vi "DCS(Upgrade).vi"(3 "error in":errorcluster) -> (10 "error out":errorcluster)   [LabVIEW 2013]
uses:
  <userlib>/Accelerator/User Interface/Controls/dcs points.ctl
  <userlib>/Accelerator/User Interface/Controls/dcs_spot.ctl
  <vilib>/gmath/NI_Gmath.lvlib
  <vilib>/Utility/miscctls.llb/LVPointTypeDef.ctl
  <vilib>/gmath/NumericalOptimization/Nonlinear Curve Fit LM.vi
  <userlib>/Accelerator/User Interface/Controls/Role ID.ctl
panel:
  in  "Waveform Path":path=path "C:/Users/Chris/Desktop/DCS(Upgrade)/Waveforms"
  in  "Nornamiled":path=path "C:/Users/Chris/Desktop/DCS(Upgrade)/dcs_data/dcs_normalized.csv"
  in  "XY and Max":path=path "C:/Users/Chris/Desktop/DCS(Upgrade)/dcs_points/dcs_points.csv"
  in  "Points to Check Noise":i32=2000
  in  "Color bar Control":cluster{dbl, u32}[](array[cluster])
  in  "stop":bool
  in  "Tab Control":T1(tab)
  out "Intensity Graph":dbl[][](graph)
  in  "Spot Save Folder":path=path "C:/Users/Chris/Desktop/DCS(Upgrade)/dcs_data"
  in  "Save Spot Image":bool
  in  "Clear Spot/Track":bool
  in  "Particle Limit":i64=500 min=0 step=10
  out "Laser spot\nMove (mm)":dbl[](array[numeric])=[nan, nan] format="%#.3g"
  out "Avg. Freq. (Hz)":dbl
  in  "Orange Cursor Position":dbl[](array[numeric])=[0.0, 0.0] min=-12.0 max=12.0 step=0.1 format="%.3g"
  out "Spot Widths":dbl[](array[numeric]) format="%.6g"
  out "Countdown to\nnext track point":i32=1
  out "XY Graph":cluster{"Y":dbl[], "Y":dbl[]}[](graph)
  in  "Load old position\nto Orange Cursor":bool
  in  "Set Orange Cursor\nto current position":bool
  out "# of Particles\nin Spot":dbl
  out "Current Spot Pos":dbl[](array[numeric])=[nan, nan] format="%.3g"
  in  "# of shots to calculate spot":i32=20
  out "Spot Size over time":dbl[][](graph)
  out "Filtered Signals":dbl[][](graph)
  out "Unfiltered Signals":ext[][](graph)
  in  "Record Normalized":bool
  in  "Record XY":bool
  in  "External Trigger":bool
  in  "Auto Threshold":bool
  out "Sampling Frequency":u16(ring) items=["40 MHz", "20 MHz", "10 MHz", "5 MHz", "2.5 MHz", "1 MHz", "100 kHz", "10 kHz"]
  out "Length of Sample":dbl caption="s" format="%^#_3g"
  out "Memory Address Pointer":ext
  out "Post trigger Size":ext
  out "Pretrigger Size":ext
  out "Trigger Generation register":i32=23 format="%.0b"
  out "status register":i8=4 format="%08b"
  out "control register":i16=23 format="%015b"
  in  "Posttrigger size":i32
  in  "Acquisition Rate":u16(ring) items=["40 MHz", "20 MHz", "10 MHz", "5 MHz", "2.5 MHz", "1 MHz", "100 kHz", "10 kHz"]
  in  "Pretrigger size":i32=1000
  in  "Rising or falling?":bool
  out "Running Errors":errorcluster
  in  "Jorger TR slot":i32=3
  in  "Timeout (# of Cycles)":i32=100
  in  "Channels":i32[](array[numeric])=[0, 1, 2, 3, 4, 5, 6, 7]
  in  "Median Filter Rank":i32=30
  in  "Thresholds":ext[](array[numeric])
  in  "Level Buffer":i32=25
  # "DAQ Parameter Indicators"
  # "DAQ Parameter Controls"
  # "Falling"
  # "Rising"
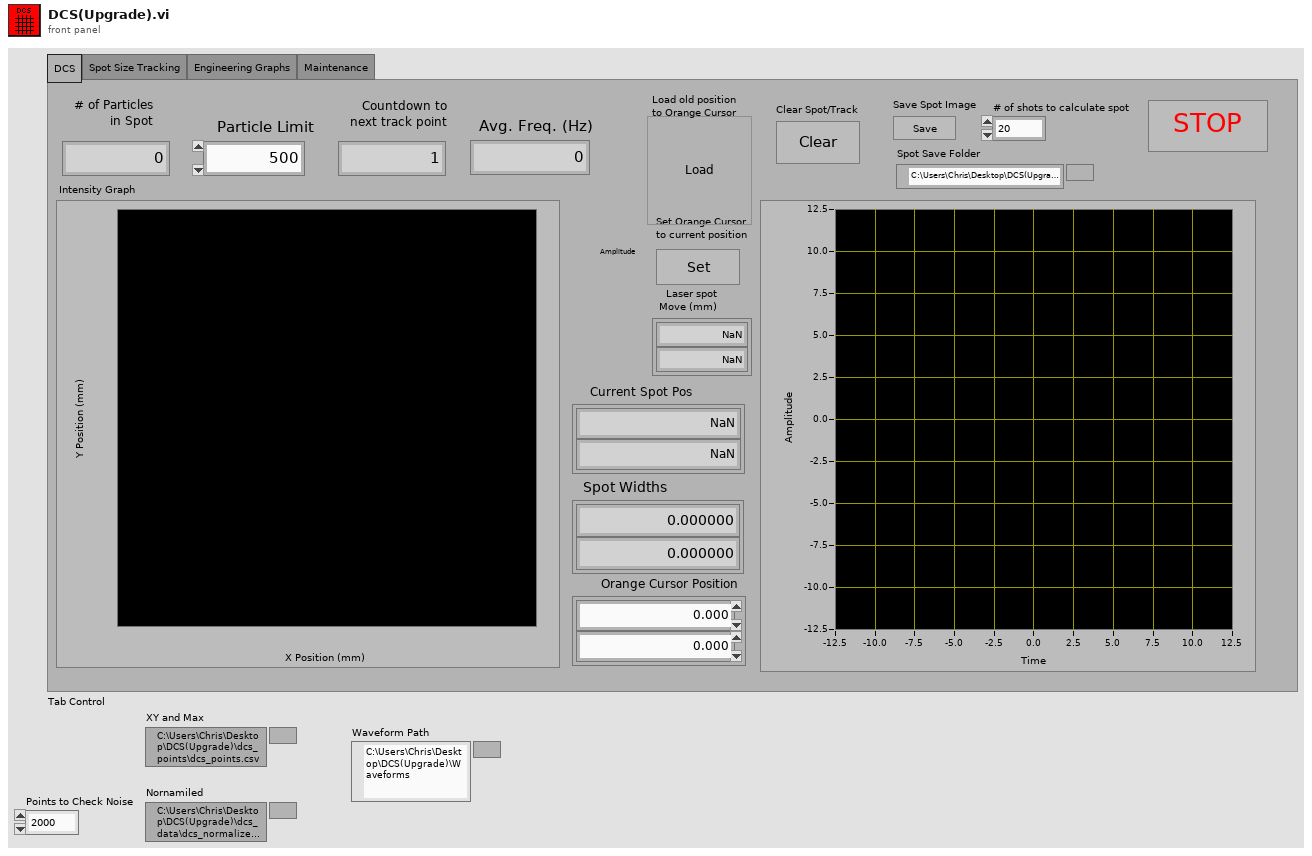
[diagram p1: front panel]
types:
  T1 = enum32{"DCS", "Spot Size Tracking", "Engineering Graphs", "Maintenance"}
  T2 = typedef "LVPointTypeDef.ctl" = cluster{"Horizontal":i16, "Vertical":i16}
  T3 = typedef "dcs_spot.ctl" = cluster{"DCS spot ID":i32, "Integer Timestamp":i64, "Spot X":dbl, "Spot Y":dbl, "Spot Width X":dbl, "Spot Width Y":dbl, "Spot Size":i32, "Experiment Settings ID":i32}
  T4 = typedef "Role ID.ctl" = enum16{"First_Detector", "Second_Detector", "Third_Detector", "LeCroy_CH1", "LeCroy_CH2", "LeCroy_CH3", "LeCroy_CH4", "PSU", "DCS 1", "DCS 2"}
  T5 = cluster{"Data":dbl[][], "Integer Timestamp":u64, "Signal Length":u32, "DCS_ID":u64, "Role ID":T4}
  T6 = typedef "dcs points.ctl" = cluster{"Integer Timestamp":i64, "X":dbl, "Y":dbl, "DCS spot ID":i32}
  T7 = cluster{"Data":dbl[][], "Integer Timestamp":u64, "Signal Length":u32, "DCS_ID":u64, "Role ID":T4}[]
  T8 = typedef "imagedata.ctl" = cluster{"image type":i32, "image depth":i32, "image":u8[], "mask":u8[], "colors":u32[], "Rectangle":cluster{"left":i16, "top":i16, "right":i16, "bottom":i16}}
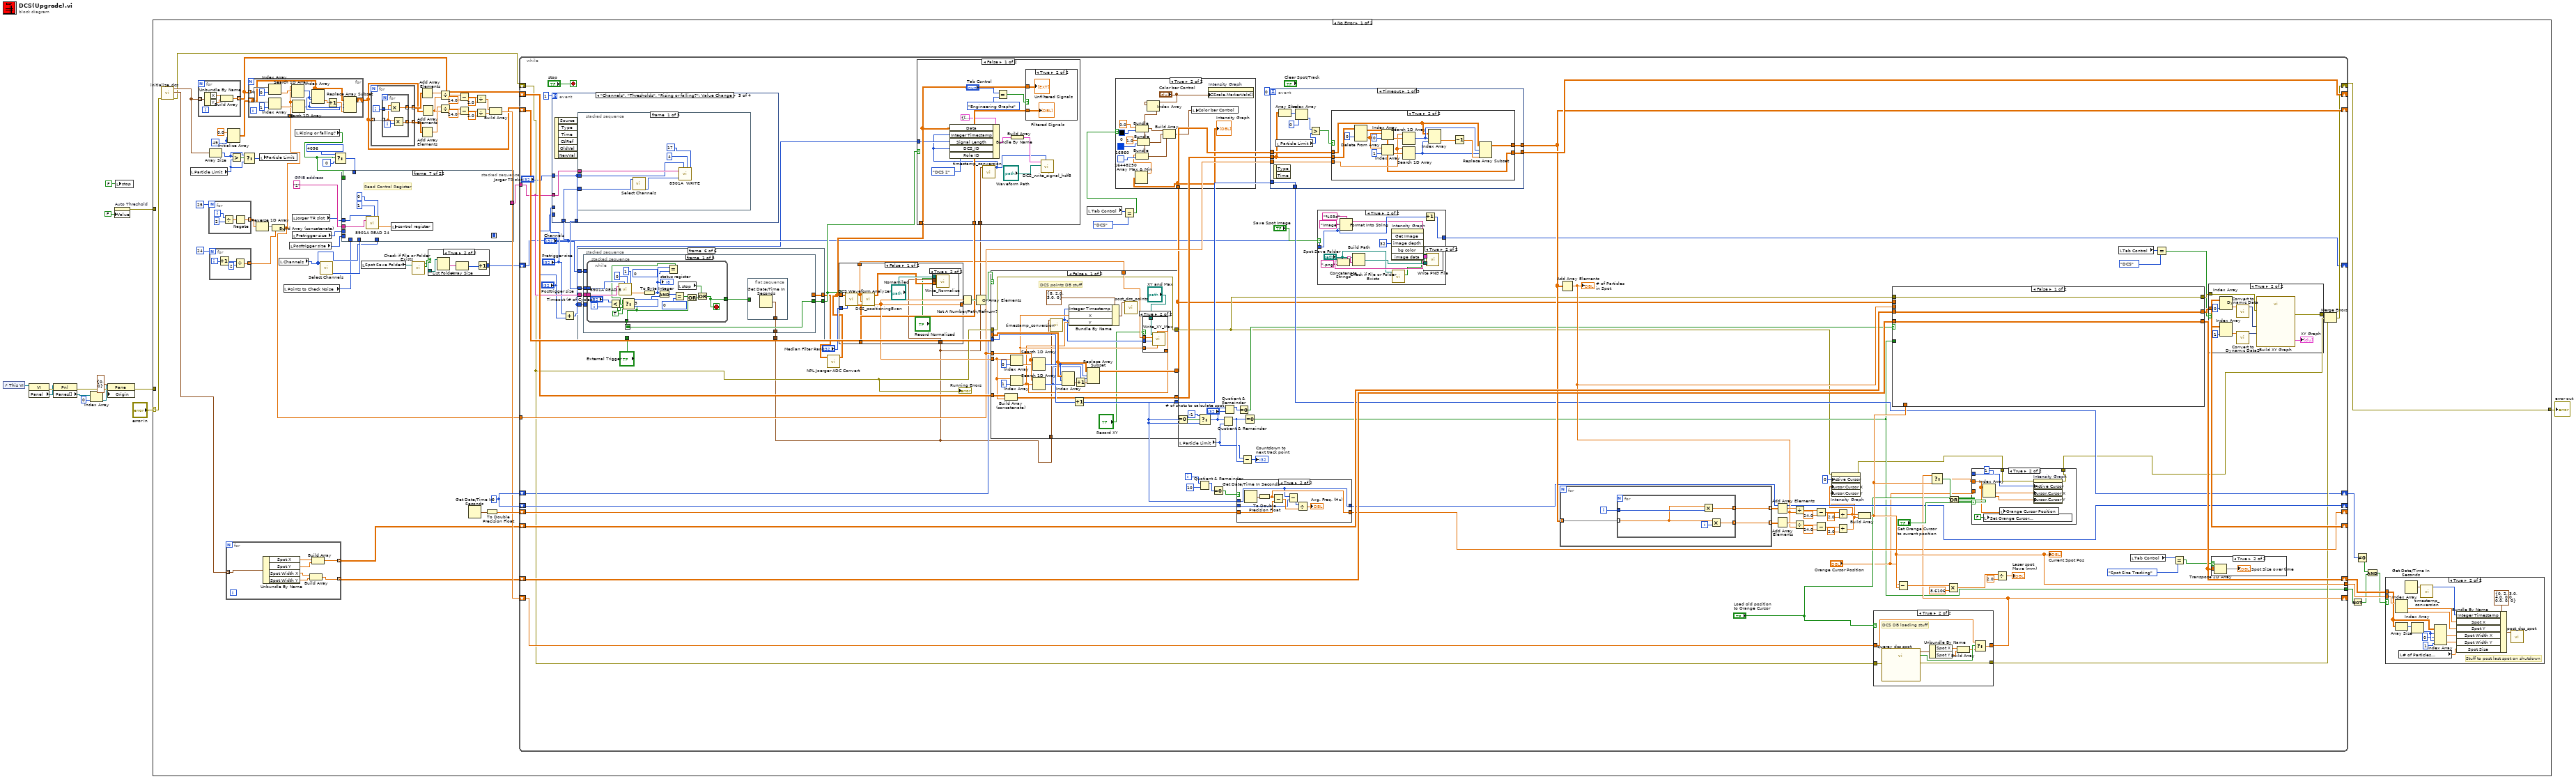
[diagram p0: block diagram]
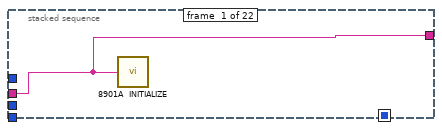
[diagram p2: hidden frame]
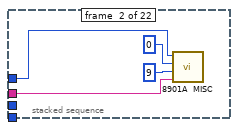
[diagram p3: hidden frame]
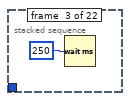
[diagram p4: hidden frame]
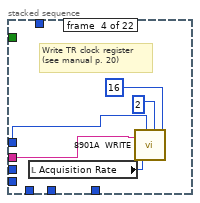
[diagram p5: hidden frame]
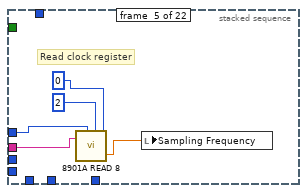
[diagram p6: hidden frame]
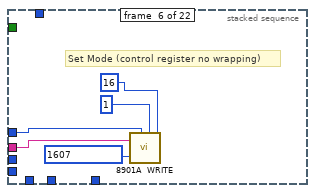
[diagram p7: hidden frame]
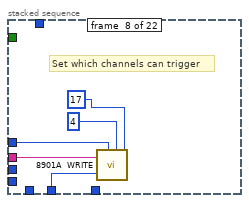
[diagram p8: hidden frame]
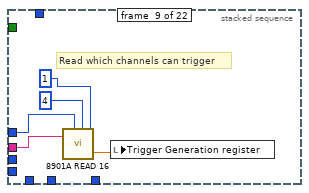
[diagram p9: hidden frame]
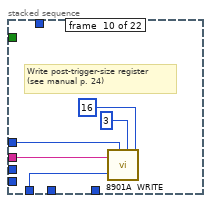
[diagram p10: hidden frame]
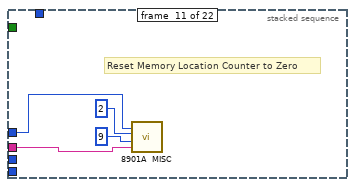
[diagram p11: hidden frame]
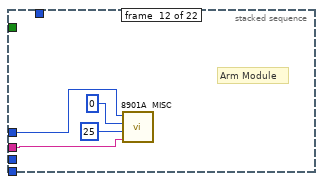
[diagram p12: hidden frame]
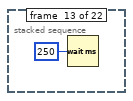
[diagram p13: hidden frame]
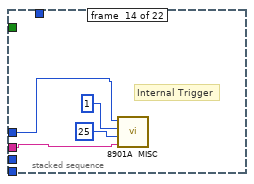
[diagram p14: hidden frame]
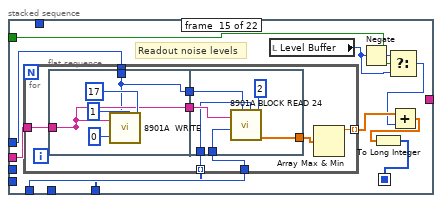
[diagram p15: hidden frame]
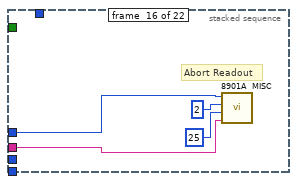
[diagram p16: hidden frame]
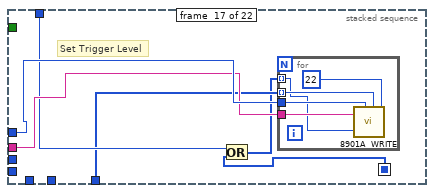
[diagram p17: hidden frame]
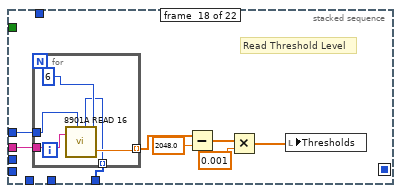
[diagram p18: hidden frame]
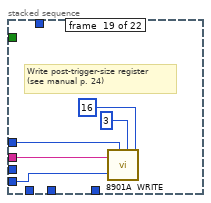
[diagram p19: hidden frame]
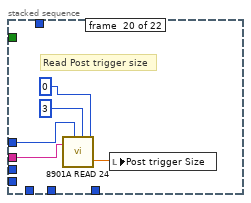
[diagram p20: hidden frame]
diagram:
  n1 = control-ref of="This VI"() -> (w11:refnum<vi>)
  n2 = property class="VI"(reference=w11) -> (error out=w10:errorcluster, "Panel"=w9:refnum<vi>)  [unwired: 1 in, 1 out]
  n3 = property class="Pnl"(reference=w9, error in=w10) -> (error out=w8:errorcluster, "Panes[]"=w7:refnum<vi>[])  [unwired: 1 out]
  n4 = Index Array(array=w7, index=0) -> (element=w5:refnum<vi>)
  n5 = property class="Pane"(reference=w5, error in=w8, "Origin"=T2 {"Horizontal"=0, "Vertical"=0}) -> (error out=w3:errorcluster)  [unwired: 1 out]
  n6 = property on="Auto Threshold" class="Bool (strict)"("Value"=FALSE ("Auto Threshold")) -> (error out=w1:errorcluster)  [unwired: 2 in, 1 out]
  n7 = local write "stop"(FALSE ("stop")) -> ()
  n8 = case shown="No Error" "error in" {
    selector: "error in" -> [w33 w956]
    tunnel: [w32 w956] -> w13
    tunnel: w3 -> [_ _]
    tunnel: w1 -> [_ _]
    frame No Error {
      w26 = "2"  # GPIB address
      w53 = 49 ("dimension size")
      w56 = 0
      n9 = call <userlib>:"initialize_dcs.vi"("error in (no error)"=w33) -> ("error out"=w27:errorcluster, "Dust Spot Array"=w45:T3[], "Dust Point Array"=w38:T6[])  [unwired: 8 in]
      n10 = local read "Particle Limit"() -> (w35:i64)
      n11 = for {
        tunnel: [w236] -> w44 mode=indexing
        tunnel: w38 -> [w235] mode=indexing
        n12 = Unbundle By Name(w235) -> ("X"=w238:dbl, "Y"=w237:dbl)
        n13 = Build Array(w238, w237) -> (w236:dbl[])
      }
      n14 = for {
        N: 25 -> [_]
        tunnel: [w267] -> w76 mode=indexing
        i -> [w270]
        n15 = Divide(x=w270, y=2) -> (x/y=w268:dbl)
        n16 = Negate(x=w268) -> (-x=w267:dbl)
      }
      n17 = Array Size(array=w38) -> (size(s)=w36:i32)
      n18 = for {
        N: 24 -> [_]
        tunnel: [w264] -> w74 mode=indexing
        i -> [w266]
        n19 = Increment(x=w266) -> (x+1=w263:i32)
        n20 = Divide(x=w263, y=2) -> (x/y=w264:dbl)
      }
      n21 = for {
        tunnel: [w230] -> w48 mode=indexing
        tunnel: [w229] -> w49 mode=indexing
        tunnel: w45 -> [w228] mode=indexing
        n22 = Unbundle By Name(w228) -> ("Spot X"=w234:dbl, "Spot Y"=w233:dbl, "Spot Width X"=w232:dbl, "Spot Width Y"=w231:dbl)
        n23 = Build Array(w232, w231) -> (w230:dbl[])
        n24 = Build Array(w234, w233) -> (w229:dbl[])
      }
      n25 = Initialize Array(0.0 ("element"), w53, w53) -> (w52:dbl[][])
      n26 = Greater?(x=w36, y=w35) -> (0:w37:bool)
      n27 = Select(t=w36, s=w37, f=w35) -> (s? t:f=w34:i64)
      n28 = Reverse 1D Array(array=w76) -> (reversed array=w75:dbl[])
      n29 = local write "Particle Limit"(w34) -> ()
      n30 = Build Array (concatenate)(w75, w74) -> (w50:dbl[])
      n31 = for {
        tunnel: w44 -> [w225] mode=indexing
        tunnel: w50 -> [w216]
        shift-right: [w217] -> w43
        shift-left: w52 -> [w218]
        n32 = Index Array(array=w225, index=0) -> (element=w224:dbl)
        n33 = Index Array(array=w225, index=1) -> (element=w223:dbl)
        n34 = Search 1D Array(1D array=w216, element=w224) -> (index of element=w220:i32)  [unwired: 1 in]
        n35 = Search 1D Array(1D array=w216, element=w223) -> (index of element=w219:i32)  [unwired: 1 in]
        n36 = Index Array(array=w218, index (row)=w220, index (col)=w219) -> (element=w222:dbl)
        n37 = Increment(x=w222) -> (x+1=w221:dbl)
        n38 = Replace Array Subset(array=w218, new element=w221, index (row)=w220, index (col)=w219) -> (w217:dbl[][])
      }
      n39 = local read "Channels"() -> (w17:i32[])
      n40 = local read "Points to Check Noise"() -> (w16:i32)
      n41 = local read "Posttrigger size"() -> (w22:i32)
      n42 = local read "Jorger TR slot"() -> (w24:i32)
      n43 = local read "Pretrigger size"() -> (w23:i32)
      n44 = local read "Rising or falling?"() -> (w15:bool)
      n45 = call <userlib>:"Select Channels.vi"("Channels"=w17) -> ("Channels in Use"=w21:u32)  [unwired: 10 in]
      n46 = Select(t=4096, s=w15, f=0) -> (s? t:f=w18:i32)
      n47 = stacked-sequence {
        seq-local: [_ _ _ _ _ _ _ _ _ _ _ _ _ _ w137 _ _ _ _ _ _ _] -> [_ _ _ _ _ _ _ _ _ _ _ _ _ _ _ _ w167 _ _ _ _ _]
        tunnel: w24 -> [_ w80 _ w87 w92 w95 w102 w106 w111 w117 w121 w124 _ w129 w139 w164 w172 w185 w193 w198 w203 w208]
        tunnel: w26 -> [w79 w81 _ w86 w91 w96 w101 w107 w112 w116 w120 w125 _ w130 w143 w163 w171 w184 w192 w197 w202 w207]
        tunnel: w23 -> [_ _ _ _ _ _ _ _ _ _ _ _ _ _ _ _ _ _ _ _ w201 _]
        tunnel: w22 -> [_ _ _ _ _ _ _ _ _ _ _ _ _ _ _ _ _ _ w191 _ _ _]
        tunnel: [w79 _ _ _ _ _ _ _ _ _ _ _ _ _ _ _ _ _ _ _ _ _] -> w25
        tunnel: w21 -> [_ _ _ _ _ _ _ w105 _ _ _ _ _ _ _ _ _ _ _ _ _ _]
        tunnel: w16 -> [_ _ _ _ _ _ _ _ _ w115 _ _ _ _ w142 _ _ _ _ _ _ _]
        tunnel: w18 -> [_ _ _ _ _ _ _ _ _ _ _ _ _ _ _ _ w170 _ _ _ _ _]
        tunnel: w17 -> [_ _ _ _ _ _ _ _ _ _ _ _ _ _ w140 _ w169 w179 _ _ _ _]
        tunnel: w15 -> [_ _ _ _ _ _ _ _ _ _ _ _ _ _ w134 _ _ _ _ _ _ _]
        frame #0 {
          n48 = call <instrlib>:"8901A  INITIALIZE.vi"("GPIB address"=w79) -> ()
        }
        frame #1 {
          n49 = call <instrlib>:"8901A  MISC.vi"("GPIB address"=w81, "f"=9, "a"=0, "n"=w80) -> ()
        }
        frame #2 {
          n50 = Wait (ms)(milliseconds to wait=250) -> ()  [unwired: 1 out]
        }
        frame #3 {
          # "Write TR clock register\n(see manual p. 20)"
          n51 = local read "Acquisition Rate"() -> (w85:u16)
          n52 = call <instrlib>:"8901A  WRITE.vi"("data"=w85, "GPIB address"=w86, "n"=w87, "a"=2, "f"=16) -> ()  [unwired: 1 in]
        }
        frame #4 {
          # "Read clock register"
          n53 = call <instrlib>:"8901A READ 8.vi"("GPIB address"=w91, "n"=w92, "a"=2, "f"=0) -> ("output"=w90:ext)  [unwired: 3 in]
          n54 = local write "Sampling Frequency"(w90) -> ()
        }
        frame #5 {
          # "Set Mode (control register no wrapping)"
          n55 = call <instrlib>:"8901A  WRITE.vi"("data"=1607, "GPIB address"=w96, "n"=w95, "a"=1, "f"=16) -> ()  [unwired: 1 in]
        }
        frame #6 {
          # "Read Control Register"
          n56 = call <instrlib>:"8901A READ 24.vi"("GPIB address"=w101, "n"=w102, "a"=1, "f"=0) -> ("output"=w100:ext)  [unwired: 3 in]
          n57 = local write "control register"(w100) -> ()
        }
        frame #7 {
          # "Set which channels can trigger"
          n58 = call <instrlib>:"8901A  WRITE.vi"("data"=w105, "GPIB address"=w107, "n"=w106, "a"=4, "f"=17) -> ()  [unwired: 1 in]
        }
        frame #8 {
          # "Read which channels can trigger"
          n59 = call <instrlib>:"8901A READ 16.vi"("GPIB address"=w112, "n"=w111, "a"=u8 4, "f"=u8 1) -> ("output"=w110:ext)  [unwired: 3 in]
          n60 = local write "Trigger Generation register"(w110) -> ()
        }
        frame #9 {
          # "Write post-trigger-size register\n(see manual p. 24)"
          n61 = call <instrlib>:"8901A  WRITE.vi"("data"=w115, "GPIB address"=w116, "n"=w117, "a"=3, "f"=16) -> ()  [unwired: 1 in]
        }
        frame #10 {
          # "Reset Memory Location Counter to Zero"
          n62 = call <instrlib>:"8901A  MISC.vi"("GPIB address"=w120, "f"=u8 9, "a"=u8 2, "n"=w121) -> ()
        }
        frame #11 {
          # "Arm Module"
          n63 = call <instrlib>:"8901A  MISC.vi"("GPIB address"=w125, "f"=25, "a"=0, "n"=w124) -> ()
        }
        frame #12 {
          n64 = Wait (ms)(milliseconds to wait=u32 250) -> ()  [unwired: 1 out]
        }
        frame #13 {
          # "Internal Trigger"
          n65 = call <instrlib>:"8901A  MISC.vi"("GPIB address"=w130, "f"=u8 25, "a"=u8 1, "n"=w129) -> ()
        }
        frame #14 {
          # "Readout noise levels"
          n66 = for {
            tunnel: w143 -> [w150]
            tunnel: w142 -> [w149]
            tunnel: [w147] -> w141 mode=indexing
            tunnel: w140 -> [w146] mode=indexing
            tunnel: w139 -> [w145]
            n67 = flat-sequence {
              tunnel: [w154] -> _
              tunnel: [w154] -> w151
              tunnel: w150 -> [w154]
              tunnel: w145 -> [w152]
              tunnel: [w152] -> w144
              tunnel: w151 -> [w161]
              tunnel: [w160] -> w148
              tunnel: w149 -> [w159]
              tunnel: w146 -> [w158]
              tunnel: w144 -> [w157]
              frame #0 {
                n68 = call <instrlib>:"8901A  WRITE.vi"("data"=0, "GPIB address"=w154, "n"=w152, "a"=1, "f"=17) -> ()  [unwired: 1 in]
              }
              frame #1 {
                n69 = call <instrlib>:"8901A BLOCK READ 24.vi"("f"=2, "a"=w158, "n"=w157, "GPIB address"=w161, "# points to read"=w159) -> ("output"=w160:ext[])  [unwired: 4 in]
              }
            }
            n70 = Array Max & Min(array=w148) -> (max value=w147:ext)  [unwired: 3 out]
          }
          n71 = local read "Level Buffer"() -> (w136:i32)
          n72 = Negate(x=w136) -> (-x=w135:i32)
          n73 = Select(t=w135, s=w134, f=w136) -> (s? t:f=w133:i32)
          n74 = Add(x=w141, y=w133) -> (x+y=w138:ext[])
          n75 = To Long Integer(number=w138) -> (32bit integer=w137:i32[])
        }
        frame #15 {
          # "Abort Readout"
          n76 = call <instrlib>:"8901A  MISC.vi"("GPIB address"=w163, "f"=25, "a"=2, "n"=w164) -> ()
        }
        frame #16 {
          # "Set Trigger Level"
          n77 = Or(x=w170, y=w167) -> (x .or. y?=w168:i32[])
          n78 = for {
            tunnel: w172 -> [w176]
            tunnel: w171 -> [w175]
            tunnel: w169 -> [w174] mode=indexing
            tunnel: w168 -> [w173] mode=indexing
            n79 = call <instrlib>:"8901A  WRITE.vi"("data"=w173, "GPIB address"=w175, "n"=w176, "a"=w174, "f"=u8 22) -> ()  [unwired: 1 in]
          }
        }
        frame #17 {
          # "Read Threshold Level"
          n80 = for {
            tunnel: w185 -> [w189]
            tunnel: w184 -> [w188]
            tunnel: [w187] -> w182 mode=indexing
            tunnel: w179 -> [w186] mode=indexing
            n81 = call <instrlib>:"8901A READ 16.vi"("GPIB address"=w188, "n"=w189, "a"=w186, "f"=u8 6) -> ("output"=w187:ext)  [unwired: 3 in]
          }
          n82 = Subtract(x=w182, y=2048.0) -> (x-y=w180:ext[])
          n83 = Multiply(x=w180, y=0.001) -> (x*y=w178:ext[])
          n84 = local write "Thresholds"(w178) -> ()
        }
        frame #18 {
          # "Write post-trigger-size register\n(see manual p. 24)"
          n85 = call <instrlib>:"8901A  WRITE.vi"("data"=w191, "GPIB address"=w192, "n"=w193, "a"=3, "f"=16) -> ()  [unwired: 1 in]
        }
        frame #19 {
          # "Read Post trigger size"
          n86 = call <instrlib>:"8901A READ 24.vi"("GPIB address"=w197, "n"=w198, "a"=3, "f"=0) -> ("output"=w196:ext)  [unwired: 3 in]
          n87 = local write "Post trigger Size"(w196) -> ()
        }
        frame #20 {
          # "Write Pretrigger size"
          n88 = call <instrlib>:"8901A  WRITE.vi"("data"=w201, "GPIB address"=w202, "n"=w203, "a"=4, "f"=16) -> ()  [unwired: 1 in]
        }
        frame #21 {
          # "Read Pretrigger size"
          n89 = call <instrlib>:"8901A READ 16.vi"("GPIB address"=w207, "n"=w208, "a"=u8 4, "f"=u8 0) -> ("output"=w206:ext)  [unwired: 3 in]
          n90 = local write "Pretrigger Size"(w206) -> ()
        }
      }
      n91 = local read "Spot Save Folder"() -> (w30:path)
      n92 = for {
        tunnel: w43 -> [w257] mode=indexing
        tunnel: [w255] -> w73 mode=indexing
        tunnel: [w254] -> w72 mode=indexing
        i -> [w256]
        n93 = for {
          tunnel: w257 -> [w259] mode=indexing
          tunnel: w256 -> [w262]
          tunnel: [w260] -> w254 mode=indexing
          tunnel: [w258] -> w255 mode=indexing
          i -> [w261]
          n94 = Multiply(x=w259, y=w262) -> (x*y=w258:dbl)
          n95 = Multiply(x=w259, y=w261) -> (x*y=w260:dbl)
        }
      }
      n96 = call <vilib>:"Check if File or Folder Exists.vi"("path"=w30) -> ("file or folder exists?"=w29:bool, "dup path"=w28:path)  [unwired: 8 in, 1 out]
      n97 = Add Array Elements(numeric array=w73) -> (sum=w71:dbl)
      n98 = Add Array Elements(numeric array=w72) -> (sum=w70:dbl)
      n99 = Add Array Elements(numeric array=w43) -> (sum=w62:dbl)
      n100 = case shown="True" w29 {
        tunnel: [0 w213] -> w31
        tunnel: w28 -> [_ w212]
        frame False {
        }
        frame True {
          n101 = List Folder(path=w212) -> (filenames=w215:string[])  [unwired: 3 in, 3 out]
          n102 = Array Size(array=w215) -> (size(s)=w214:i32)
          n103 = Increment(x=w214) -> (x+1=w213:i32)
        }
      }
      n104 = Divide(x=w71, y=w62) -> (x/y=w69:dbl)
      n105 = Divide(x=w70, y=w62) -> (x/y=w68:dbl)
      n106 = Subtract(x=w69, y=24.0) -> (x-y=w60:dbl)
      n107 = Subtract(x=w68, y=24.0) -> (x-y=w66:dbl)
      n108 = Get Date/Time In Seconds() -> (seconds since 1Jan1904=w58:timestamp)
      n109 = Divide(x=w60, y=2.0) -> (x/y=w59:dbl)
      n110 = Divide(x=w66, y=2.0) -> (x/y=w63:dbl)
      n111 = To Double Precision Float(number=w58) -> (double precision float=w57:dbl)
      n112 = Build Array(w59, w63) -> (w51:dbl[])
      n113 = while {
        shift-right: [w349] -> _
        shift-left: w44 -> [w351]
        shift-right: [w334] -> _
        shift-left: w43 -> [w373]
        tunnel: w50 -> [w325]
        shift-right: [w333] -> _
        shift-left: w51 -> [w361]
        tunnel: [w348] -> w55
        shift-right: [w324] -> w32
        shift-left: w27 -> [w286]
        shift-right: [w346] -> _
        shift-left: w49 -> [w338]
        shift-right: [w318] -> w42
        shift-left: w56 -> [w273]
        shift-right: [w347] -> w46
        shift-left: w48 -> [w350]
        shift-right: [w331] -> _
        shift-left: w57 -> [w345]
        shift-right: [w330] -> _
        shift-left: w56 -> [w332]
        tunnel: [w315] -> w47
        shift-right: [w275] -> _
        shift-left: w31 -> [w274]
        tunnel: w25 -> [w290]
        i -> [w301]
        stop <- "stop" stop-if-true
        n114 = event shown="[2] \"Channels\", \"Thresholds\", \"Rising or falling?\": Value Change" {
          selector: _ -> [_ _ _ _]
          dyn-events: _ -> [_ _ _ _]
          timeout: 1 -> [_ _ _ _]
          tunnel: w290 -> [_ w525 w590 w626]
          tunnel: "Pretrigger size" -> [_ w524 _ _]
          tunnel: "Posttrigger size" -> [_ w523 _ w621]
          tunnel: [w512 w513 w589 w623] -> w289
          tunnel: "Channels" -> [_ w515 w588 w624]
          tunnel: "Jorger TR slot" -> [_ w513 w589 w623]
          event Timeout {
            n115 = event-data() -> ()  [unwired: 1 in, 3 out]
            n116 = local read "Jorger TR slot"() -> (w512:i32)
          }
          event "Acquisition Rate", "Pretrigger size", "Posttrigger size": Value Change {
            n117 = event-data() -> ()  [unwired: 1 in, 6 out]
            n118 = local read "Acquisition Rate"() -> (w522:u16)
            n119 = call <userlib>:"Select Channels.vi"("Channels"=w515) -> ("Channels in Use"=w514:u32)  [unwired: 10 in]
            n120 = stacked-sequence {
              tunnel: w513 -> [w560 w565 w570 w575 w580 w585]
              tunnel: w525 -> [w559 w564 w569 w574 w579 w584]
              tunnel: w524 -> [_ _ _ _ w578 _]
              tunnel: w523 -> [w558 _ _ _ _ _]
              tunnel: w514 -> [_ _ _ _ _ _]
              frame #0 {
                # "Write post-trigger-size register\n(see manual p. 24)"
                n121 = call <instrlib>:"8901A  WRITE.vi"("data"=w558, "GPIB address"=w559, "n"=w560, "a"=3, "f"=16) -> ()  [unwired: 1 in]
              }
              frame #1 {
                # "Read Post trigger size"
                n122 = call <instrlib>:"8901A READ 24.vi"("GPIB address"=w564, "n"=w565, "a"=3, "f"=0) -> ("output"=→"Post trigger Size":ext)  [unwired: 3 in]
              }
              frame #2 {
                # "Write TR clock register\n(see manual p. 20)"
                n123 = call <instrlib>:"8901A  WRITE.vi"("data"="Acquisition Rate", "GPIB address"=w569, "n"=w570, "a"=2, "f"=16) -> ()  [unwired: 1 in]
              }
              frame #3 {
                # "Read clock register"
                n124 = call <instrlib>:"8901A READ 8.vi"("GPIB address"=w574, "n"=w575, "a"=2, "f"=0) -> ("output"=→"Sampling Frequency":ext)  [unwired: 3 in]
              }
              frame #4 {
                # "Write Pretrigger size"
                n125 = call <instrlib>:"8901A  WRITE.vi"("data"=w578, "GPIB address"=w579, "n"=w580, "a"=4, "f"=16) -> ()  [unwired: 1 in]
              }
              frame #5 {
                # "Read Pretrigger size"
                n126 = call <instrlib>:"8901A READ 16.vi"("GPIB address"=w584, "n"=w585, "a"=u8 4, "f"=u8 0) -> ("output"=→"Pretrigger Size":ext)  [unwired: 3 in]
              }
            }
            n127 = case shown="0, Default" w522 {
              tunnel: [w526 w530 w534 w538 w542 w546 w550 w554] -> w520
              frame 0, Default {
                n128 = Power Of 10(x=6) -> (10^x=w528:dbl)
                n129 = Multiply(x=40, y=w528) -> (x*y=w526:dbl)
              }
              frame 1 {
                n130 = Power Of 10(x=6) -> (10^x=w532:dbl)
                n131 = Multiply(x=20, y=w532) -> (x*y=w530:dbl)
              }
              frame 2 {
                n132 = Power Of 10(x=6) -> (10^x=w536:dbl)
                n133 = Multiply(x=10, y=w536) -> (x*y=w534:dbl)
              }
              frame 3 {
                n134 = Power Of 10(x=6) -> (10^x=w540:dbl)
                n135 = Multiply(x=5, y=w540) -> (x*y=w538:dbl)
              }
              frame 4 {
                n136 = Power Of 10(x=6) -> (10^x=w544:dbl)
                n137 = Multiply(x=2.5, y=w544) -> (x*y=w542:dbl)
              }
              frame 5 {
                n138 = Power Of 10(x=6) -> (10^x=w548:dbl)
                n139 = Multiply(x=1, y=w548) -> (x*y=w546:dbl)
              }
              frame 6 {
                n140 = Power Of 10(x=3) -> (10^x=w552:dbl)
                n141 = Multiply(x=100, y=w552) -> (x*y=w550:dbl)
              }
              frame 7 {
                n142 = Power Of 10(x=3) -> (10^x=w556:dbl)
                n143 = Multiply(x=10, y=w556) -> (x*y=w554:dbl)
              }
            }
            n144 = local read "Posttrigger size"() -> (w519:i32)
            n145 = Reciprocal(x=w520) -> (1/x=w521:dbl)
            n146 = local read "Pretrigger size"() -> (w518:i32)
            n147 = Add(x=w519, y=w518) -> (x+y=w517:i32)
            n148 = Multiply(x=w517, y=w521) -> (x*y=→"Length of Sample":dbl)
          }
          event "Channels", "Thresholds", "Rising or falling?": Value Change {
            n149 = event-data() -> ()  [unwired: 1 in, 6 out]
            n150 = stacked-sequence {
              tunnel: w590 -> [w594 w598 w606]
              tunnel: w589 -> [w593 w599 w605]
              tunnel: w588 -> [w591 _ w604]
              frame #0 {
                n151 = call <userlib>:"Select Channels.vi"("Channels"=w591) -> ("Channels in Use"=w592:u32)  [unwired: 10 in]
                n152 = call <instrlib>:"8901A  WRITE.vi"("data"=w592, "GPIB address"=w594, "n"=w593, "a"=4, "f"=17) -> ()  [unwired: 1 in]
              }
              frame #1 {
                n153 = call <instrlib>:"8901A READ 16.vi"("GPIB address"=w598, "n"=w599, "a"=u8 4, "f"=u8 1) -> ("output"=→"Trigger Generation register":ext)  [unwired: 3 in]
              }
              frame #2 {
                n154 = Add(x="Thresholds", y=2.048) -> (x+y=w614:ext[])
                n155 = Multiply(x=w614, y=1000.0) -> (x*y=w612:ext[])
                n156 = Select(t=4096, s="Rising or falling?", f=0) -> (s? t:f=w608:i32)
                n157 = To Long Integer(number=w612) -> (32bit integer=w609:i32[])
                n158 = Or(x=w608, y=w609) -> (x .or. y?=w607:i32[])
                n159 = for {
                  tunnel: w605 -> [w619]
                  tunnel: w606 -> [w618]
                  tunnel: w604 -> [w617] mode=indexing
                  tunnel: w607 -> [w616] mode=indexing
                  n160 = call <instrlib>:"8901A  WRITE.vi"("data"=w616, "GPIB address"=w618, "n"=w619, "a"=w617, "f"=u8 22) -> ()  [unwired: 1 in]
                }
              }
            }
          }
          event "Auto Threshold": Value Change {
            n161 = event-data() -> ()  [unwired: 1 in, 6 out]
            n162 = stacked-sequence {
              seq-local: [_ _ _ _ _ _ _ w656 _ _ _ _] -> [_ _ _ _ _ _ _ _ _ w689 _ _]
              tunnel: w626 -> [w629 w633 w637 w641 w645 _ w650 w660 w684 w691 w704 w717]
              tunnel: "Points to Check Noise" -> [w628 _ _ _ _ _ _ w658 _ _ _ _]
              tunnel: w623 -> [w627 w632 w638 w642 w646 _ w651 w659 w685 w690 w703 w716]
              tunnel: w624 -> [_ _ _ _ _ _ _ w657 _ w692 w705 _]
              tunnel: w621 -> [_ _ _ _ _ _ _ _ _ _ _ w715]
              frame #0 {
                # "Write post-trigger-size register\n(see manual p. 24)"
                n163 = call <instrlib>:"8901A  WRITE.vi"("data"=w628, "GPIB address"=w629, "n"=w627, "a"=3, "f"=16) -> ()  [unwired: 1 in]
              }
              frame #1 {
                # "Turn off Wrapping"
                n164 = call <instrlib>:"8901A  WRITE.vi"("data"=1607, "GPIB address"=w633, "n"=w632, "a"=1, "f"=16) -> ()  [unwired: 1 in]
              }
              frame #2 {
                # "Reset Memory Counter to Zero"
                n165 = call <instrlib>:"8901A  MISC.vi"("GPIB address"=w637, "f"=u8 9, "a"=u8 2, "n"=w638) -> ()
              }
              frame #3 {
                # "Arm Module"
                n166 = call <instrlib>:"8901A  MISC.vi"("GPIB address"=w641, "f"=25, "a"=0, "n"=w642) -> ()
              }
              frame #4 {
                n167 = call <instrlib>:"8901A  MISC.vi"("GPIB address"=w645, "f"=u8 21, "a"=u8 2, "n"=w646) -> ()
              }
              frame #5 {
                n168 = Wait (ms)(milliseconds to wait=u32 250) -> ()  [unwired: 1 out]
              }
              frame #6 {
                # "Internal Trigger"
                n169 = call <instrlib>:"8901A  MISC.vi"("GPIB address"=w650, "f"=u8 25, "a"=u8 1, "n"=w651) -> ()
              }
              frame #7 {
                n170 = for {
                  tunnel: w660 -> [w671]
                  tunnel: w658 -> [w670]
                  tunnel: [w668] -> w664 mode=indexing
                  tunnel: w657 -> [w667] mode=indexing
                  tunnel: w659 -> [w666]
                  n171 = flat-sequence {
                    tunnel: [w675] -> _
                    tunnel: [w675] -> w672
                    tunnel: w671 -> [w675]
                    tunnel: w666 -> [w673]
                    tunnel: [w673] -> w665
                    tunnel: w672 -> [w682]
                    tunnel: [w681] -> w669
                    tunnel: w670 -> [w680]
                    tunnel: w667 -> [w679]
                    tunnel: w665 -> [w678]
                    frame #0 {
                      n172 = call <instrlib>:"8901A  WRITE.vi"("data"=0, "GPIB address"=w675, "n"=w673, "a"=1, "f"=17) -> ()  [unwired: 1 in]
                    }
                    frame #1 {
                      n173 = call <instrlib>:"8901A BLOCK READ 24.vi"("f"=2, "a"=w679, "n"=w678, "GPIB address"=w682, "# points to read"=w680) -> ("output"=w681:ext[])  [unwired: 4 in]
                    }
                  }
                  n174 = Array Max & Min(array=w669) -> (max value=w668:ext)  [unwired: 3 out]
                }
                n175 = local read "Rising or falling?"() -> (w654:bool)
                n176 = Negate(x="Level Buffer") -> (-x=w662:i32)
                n177 = Select(t=w662, s=w654, f="Level Buffer") -> (s? t:f=w661:i32)
                n178 = Add(x=w664, y=w661) -> (x+y=w663:ext[])
                n179 = To Long Integer(number=w663) -> (32bit integer=w656:i32[])
              }
              frame #8 {
                # "Abort Readout"
                n180 = call <instrlib>:"8901A  MISC.vi"("GPIB address"=w684, "f"=25, "a"=2, "n"=w685) -> ()
              }
              frame #9 {
                n181 = local read "Rising or falling?"() -> (w688:bool)
                n182 = Select(t=4096, s=w688, f=0) -> (s? t:f=w693:i32)
                n183 = Or(x=w693, y=w689) -> (x .or. y?=w696:i32[])
                n184 = for {
                  tunnel: w690 -> [w700]
                  tunnel: w691 -> [w699]
                  tunnel: w692 -> [w698] mode=indexing
                  tunnel: w696 -> [w697] mode=indexing
                  n185 = call <instrlib>:"8901A  WRITE.vi"("data"=w697, "GPIB address"=w699, "n"=w700, "a"=w698, "f"=u8 22) -> ()  [unwired: 1 in]
                }
              }
              frame #10 {
                n186 = for {
                  tunnel: w703 -> [w713]
                  tunnel: w704 -> [w712]
                  tunnel: [w711] -> w706 mode=indexing
                  tunnel: w705 -> [w710] mode=indexing
                  n187 = call <instrlib>:"8901A READ 16.vi"("GPIB address"=w712, "n"=w713, "a"=w710, "f"=u8 6) -> ("output"=w711:ext)  [unwired: 3 in]
                }
                n188 = Subtract(x=w706, y=2048.0) -> (x-y=w707:ext[])
                n189 = Multiply(x=w707, y=0.001) -> (x*y=w702:ext[])
                n190 = local write "Thresholds"(w702) -> ()
              }
              frame #11 {
                # "Write post-trigger-size register\n(see manual p. 24)"
                n191 = call <instrlib>:"8901A  WRITE.vi"("data"=w715, "GPIB address"=w717, "n"=w716, "a"=3, "f"=16) -> ()  [unwired: 1 in]
              }
            }
            n192 = local write "Auto Threshold"(FALSE ("Auto Threshold")) -> ()
          }
        }
        n193 = Add(x="Pretrigger size", y="Posttrigger size") -> (x+y=w272:i32)
        n194 = stacked-sequence {
          tunnel: w289 -> [w406 w413 w417 w420 w424 w433]
          tunnel: w290 -> [w405 w412 w416 w421 w425 w434]
          tunnel: [_ _ _ _ _ w432] -> w283
          tunnel: w272 -> [_ _ _ _ _ w431]
          tunnel: "Channels" -> [_ _ _ _ _ w430]
          tunnel: [_ _ _ _ _ w429] -> w280
          tunnel: "External Trigger" -> [w403 _ _ _ _ _]
          tunnel: [_ _ _ _ _ w428] -> w271
          frame #0 {
            # "Set Control Register"
            n195 = case shown="True" w403 {
              tunnel: [1615 79 ("data")] -> w404
              frame False {
              }
              frame True {
              }
            }
            n196 = call <instrlib>:"8901A  WRITE.vi"("data"=w404, "GPIB address"=w405, "n"=w406, "a"=1, "f"=16) -> ()  [unwired: 1 in]
          }
          frame #1 {
            # "Read Control Register"
            n197 = call <instrlib>:"8901A READ 24.vi"("GPIB address"=w412, "n"=w413, "a"=1, "f"=0) -> ("output"=→"control register":ext)  [unwired: 3 in]
          }
          frame #2 {
            # "Reset Memory Location counter to 0"
            n198 = call <instrlib>:"8901A  MISC.vi"("GPIB address"=w416, "f"=u8 9, "a"=u8 2, "n"=w417) -> ()
          }
          frame #3 {
            # "Arm Module"
            n199 = call <instrlib>:"8901A  MISC.vi"("GPIB address"=w421, "f"=25, "a"=0, "n"=w420) -> ()
          }
          frame #4 {
            # "Clear All Valid Trigger tags"
            n200 = call <instrlib>:"8901A  MISC.vi"("GPIB address"=w425, "f"=u8 21, "a"=u8 2, "n"=w424) -> ()
          }
          frame #5 {
            n201 = stacked-sequence {
              seq-local: [w437 _ _ _ _] -> [_ w463 w474 _ _]
              tunnel: w434 -> [w439 w461 w471 w503 w508]
              tunnel: w433 -> [w438 w462 w470 w504 w509]
              tunnel: [w437 _ _ _ _] -> w432
              tunnel: w431 -> [_ _ w473 _ _]
              tunnel: w430 -> [_ _ w472 _ _]
              tunnel: [_ _ w469 _ _] -> w429
              tunnel: [w435 _ _ _ _] -> w428
              frame #0 {
                n202 = while {
                  tunnel: w439 -> [w453]
                  tunnel: w438 -> [w452]
                  tunnel: [w442] -> w437
                  tunnel: [w441] -> w436
                  i -> [w451]
                  stop <- w441 stop-if-true
                  n203 = Less?(x="Timeout (# of Cycles)", y=w451) -> (x < y?=w444:bool)
                  n204 = call <instrlib>:"8901A READ 8.vi"("GPIB address"=w453, "n"=w452, "a"=0, "f"=1) -> ("output"=w456:ext)  [unwired: 3 in]
                  n205 = To Byte Integer(number=w456) -> (8bit integer=w447:i8)
                  "status register" <- w447
                  n206 = And(x=w447, y=i8 3) -> (x .and. y?=w457:i8)
                  n207 = Equal?(x=w447, y=i8 0) -> (x = y?=w445:bool)
                  n208 = Select(t=TRUE, s=w445, f=w444) -> (s? t:f=w442:bool)
                  n209 = Equal?(x=w457, y=i8 0) -> (x = y?=w449:bool)
                  n210 = local read "stop"() -> (w448:bool)
                  n211 = Or(x=w449, y=w442) -> (x .or. y?=w458:bool)
                  n212 = Or(x=w448, y=w458) -> (x .or. y?=w441:bool)
                }
                n213 = flat-sequence {
                  tunnel: w436 -> [_]
                  tunnel: [w440] -> w435
                  frame #0 {
                    n214 = Get Date/Time In Seconds() -> (seconds since 1Jan1904=w440:timestamp)
                  }
                }
              }
              frame #1 {
                n215 = case shown="False" w463 {
                  tunnel: w462 -> [w466 _]
                  tunnel: w461 -> [w465 _]
                  frame False {
                    n216 = call <instrlib>:"8901A READ 24.vi"("GPIB address"=w465, "n"=w466, "a"=u8 9, "f"=u8 0) -> ("output"=→"Memory Address Pointer":ext)  [unwired: 3 in]
                  }
                  frame True {
                  }
                }
              }
              frame #2 {
                n217 = case shown="False" w474 {
                  tunnel: w473 -> [w479 _]
                  tunnel: w472 -> [w480 _]
                  tunnel: w471 -> [w478 _]
                  tunnel: w470 -> [w477 _]
                  tunnel: [w475 ext[][] [[nan]] ("output")] -> w469
                  frame False {
                    n218 = local read "Memory Address Pointer"() -> (w476:ext)
                    n219 = for {
                      N: 8 -> [_]
                      tunnel: w480 -> [w484] mode=indexing
                      tunnel: w479 -> [w483]
                      tunnel: w478 -> [w488]
                      tunnel: w477 -> [w487]
                      tunnel: w476 -> [w490]
                      tunnel: [w482] -> w475 mode=indexing
                      n220 = Subtract(x=w490, y=w483) -> (x-y=w489:ext)
                      n221 = flat-sequence {
                        tunnel: w489 -> [w493]
                        tunnel: w488 -> [w491]
                        tunnel: w487 -> [w492]
                        tunnel: [w492] -> w486
                        tunnel: [w491] -> w485
                        tunnel: w486 -> [w499]
                        tunnel: w485 -> [w498]
                        tunnel: w484 -> [w500]
                        tunnel: w483 -> [w497]
                        tunnel: [w496] -> w482
                        frame #0 {
                          n222 = call <instrlib>:"8901A  WRITE.vi"("data"=w493, "GPIB address"=w491, "n"=w492, "a"=1, "f"=17) -> ()  [unwired: 1 in]
                        }
                        frame #1 {
                          n223 = call <instrlib>:"8901A BLOCK READ 24.vi"("f"=2, "a"=w500, "n"=w499, "GPIB address"=w498, "# points to read"=w497) -> ("output"=w496:ext[])  [unwired: 4 in]
                        }
                      }
                    }
                  }
                  frame True {
                  }
                }
              }
              frame #3 {
                # "Abort Readout"
                n224 = call <instrlib>:"8901A  MISC.vi"("GPIB address"=w503, "f"=25, "a"=2, "n"=w504) -> ()
              }
              frame #4 {
                # "Read in control register"
                n225 = call <instrlib>:"8901A READ 24.vi"("GPIB address"=w508, "n"=w509, "a"=1, "f"=0) -> ("output"=w507:ext)  [unwired: 3 in]
                n226 = local write "control register"(w507) -> ()
              }
            }
          }
        }
        n227 = call <userlib>:"NPL Joerger ADC Convert.vi"("Input"=w280) -> ("Output"=w279:ext[][])  [unwired: 10 in]
        n228 = case shown="False" w283 {
          tunnel: [w397 w401] -> w358
          tunnel: w279 -> [w396 _]
          tunnel: "Median Filter Rank" -> [w395 _]
          tunnel: [w394 dbl[][] [] ("Filtered Signals")] -> w284
          tunnel: [w393 w401] -> w277
          tunnel: w271 -> [w390 _]
          frame False {
            n229 = call <userlib>:"DCS Waveform Analyzer.vi"("Rank"=w395, "8 DCS Waveforms"=w396) -> ("Filtered Signals"=w394:dbl[][], "Maxs"=w393:dbl[])  [unwired: 8 in]
            n230 = call <userlib>:"DCS_positioningEvan.vi"("Data"=w393) -> ("X-Y position"=w397:dbl[], "Normalized Data"=w391:dbl[][])  [unwired: 9 in]
            n231 = case shown="True" "Record Normalized" {
              tunnel: "Nornamiled" -> [_ w400]
              tunnel: w391 -> [_ w399]
              tunnel: w390 -> [_ w398]
              frame False {
              }
              frame True {
                n232 = call <userlib>:"Write_Normalize.vi"("Normalized Data"=w399, "seconds since 1Jan1904"=w398, "Nornamiled"=w400) -> ()  [unwired: 9 in]
              }
            }
          }
          frame True {
            w401 = dbl[] [nan] ("X-Y position")
          }
        }
        n233 = case shown="False" w283 {
          tunnel: w279 -> [w381 _]
          tunnel: w284 -> [w386 _]
          tunnel: w271 -> [w380 _]
          tunnel: w272 -> [w375 _]
          frame False {
            n234 = call <userlib>:"timestamp_conversion.vi"("Time Stamp"=w380) -> ("Integer Time"=w374:i64)  [unwired: 8 in, 1 out]
            n235 = Bundle By Name(cluster=T5 {"Data"=[], "Integer Timestamp"=0, "Signal Length"=0, "DCS_ID"=0, "Role ID"=enum."First_Detector"} ("Cluster"), "Data"=w381, "Integer Timestamp"=w374, "Signal Length"=w375, "DCS_ID"=w374, "Role ID"=Role_ID."DCS 2") -> (w384:T5)
            n236 = Equal?(x="Tab Control", y=T1."Engineering Graphs") -> (x = y?=w376:bool)
            n237 = Build Array(w384) -> (w383:T7)
            n238 = case shown="True" w376 {
              tunnel: w386 -> [_ w388]
              tunnel: w381 -> [_ w387]
              frame False {
              }
              frame True {
                "Filtered Signals" <- w388
                "Unfiltered Signals" <- w387
              }
            }
            n239 = call <userlib>:"DCS_write_signal_hdf5.vi"("Index"=w374, "Save Path"="Waveform Path", "Signal array"=w383) -> ()  [unwired: 8 in, 1 out]
          }
          frame True {
          }
        }
        n240 = Not A Number/Path/Refnum?(number/path/refnum=w358) -> (NaN/Path/Refnum?=w372:bool[])
        n241 = Or Array Elements(Boolean array=w372) -> (logical OR=w357:bool)
        n242 = case shown="False" w357 {
          tunnel: w373 -> [w944 w955]
          tunnel: [w939 w955] -> w302
          tunnel: w325 -> [w938 _]
          tunnel: w358 -> [w934 _]
          tunnel: w273 -> [w937 w954]
          tunnel: [w936 w954] -> w319
          tunnel: w351 -> [w935 w953]
          tunnel: [w933 w953] -> w328
          tunnel: w286 -> [w926 w952]
          tunnel: [w926 w952] -> w307
          tunnel: w277 -> [w927 _]
          tunnel: w271 -> [w924 _]
          frame False {
            # "DCS points DB stuff"
            n243 = Build Array (concatenate)(w935, w934) -> (w933:dbl[][])
            n244 = Index Array(array=w934, index=0) -> (element=w930:dbl)
            n245 = Index Array(array=w934, index=1) -> (element=w929:dbl)
            n246 = Search 1D Array(1D array=w938, element=w930) -> (index of element=w943:i32)  [unwired: 1 in]
            n247 = Search 1D Array(1D array=w938, element=w929) -> (index of element=w942:i32)  [unwired: 1 in]
            n248 = call <userlib>:"timestamp_conversion.vi"("Time Stamp"=w924) -> ("Integer Time"=w925:i64)  [unwired: 8 in, 1 out]
            n249 = Index Array(array=w944, index (row)=w943, index (col)=w942) -> (element=w941:dbl)
            n250 = Bundle By Name(cluster=T6 {"Integer Timestamp"=8, "X"=2.0, "Y"=3.0, "DCS spot ID"=0} ("DCS points"), "Integer Timestamp"=w925, "X"=w930, "Y"=w929) -> (w932:T6)
            n251 = Increment(x=w937) -> (x+1=w936:i32)
            n252 = Increment(x=w941) -> (x+1=w940:dbl)
            n253 = Replace Array Subset(array=w944, new element=w940, index (row)=w943, index (col)=w942) -> (w939:dbl[][])
            n254 = call <userlib>:"post_dcs_points.vi"("DCS points"=w932) -> ()  [unwired: 10 in, 1 out]
            n255 = case shown="True" "Record XY" {
              tunnel: w930 -> [_ w951]
              tunnel: w929 -> [_ w950]
              tunnel: "XY and Max" -> [_ w949]
              tunnel: w927 -> [_ w948]
              tunnel: w925 -> [_ w947]
              frame False {
              }
              frame True {
                n256 = call <userlib>:"Write_XY_Max.vi"("Numeric 2"=w951, "Numeric"=w950, "Integer Time"=w947, "X-Y position"=w948, "XY and Max"=w949) -> ()  [unwired: 7 in]
              }
            }
          }
          frame True {
          }
        }
        n257 = local read "Tab Control"() -> (w294:T1)
        n258 = Equal?(x=w294, y=T1."DCS") -> (x = y?=w292:bool)
        n259 = case shown="True" w292 {
          tunnel: w302 -> [_ w722]
          frame False {
          }
          frame True {
            n260 = Array Max & Min(array=w722) -> (max value=w721:dbl)  [unwired: 3 out]
            n261 = Index Array(array="Color bar Control") -> (element=w730:cluster{dbl, u32})  [unwired: 1 in]
            n262 = Bundle(cluster=w730, 0.0, u32 0) -> (w731:cluster{dbl, u32})
            n263 = Bundle(cluster=w730, w721, u32 16448250) -> (w728:cluster{dbl, u32})
            n264 = Bundle(cluster=w730, 1.0, u32 16860) -> (w729:cluster{dbl, u32})
            n265 = Build Array(w731, w729, w728) -> (w720:cluster{dbl, u32}[])
            n266 = local write "Color bar Control"(w720) -> ()
            n267 = property on="Intensity Graph" class="IntGraph (strict)"("ZScale.MarkerVals[]"="Color bar Control") -> ()  [unwired: 2 in, 2 out]
            "Intensity Graph" <- w722
          }
        }
        n268 = Equal To 0?(x=w319) -> (x = 0?=w355:bool)
        n269 = local read "Particle Limit"() -> (w323:i64)
        n270 = Select(t=-1, s=w355, f=w319) -> (s? t:f=w322:i32)
        n271 = Quotient & Remainder(x=w301, y=10) -> (x-y*floor(x/y)=w344:i32)  [unwired: 1 out]
        n272 = Equal To 0?(x=w344) -> (x = 0?=w299:bool)
        n273 = Quotient & Remainder(x=w322, y=w323) -> (x-y*floor(x/y)=w353:i64)  [unwired: 1 out]
        n274 = Quotient & Remainder(x=w322, y="# of shots to calculate spot") -> (x-y*floor(x/y)=w321:i32)  [unwired: 1 out]
        n275 = case shown="True" w299 {
          tunnel: w345 -> [w844 w851]
          tunnel: [w844 w848] -> w331
          tunnel: [w843 w847] -> w330
          tunnel: w332 -> [w843 w846]
          tunnel: w319 -> [_ w847]
          frame False {
          }
          frame True {
            n276 = Get Date/Time In Seconds() -> (seconds since 1Jan1904=w852:timestamp)
            n277 = To Double Precision Float(number=w852) -> (double precision float=w848:dbl)
            n278 = Subtract(x=w848, y=w851) -> (x-y=w850:dbl)
            n279 = Subtract(x=w847, y=w846) -> (x-y=w845:i32)
            n280 = Divide(x=w845, y=w850) -> (x/y=→"Avg. Freq. (Hz)":dbl)
          }
        }
        n281 = Equal To 0?(x=w321) -> (x = 0?=w314:bool)
        n282 = Subtract(x=w323, y=w353) -> (x-y=→"Countdown to\nnext track point":i64)
        n283 = Equal To 0?(x=w353) -> (x = 0?=w315:bool)
        n284 = event shown="[0] Timeout" {
          selector: _ -> [_ _ _]
          dyn-events: _ -> [_ _ _]
          timeout: 0 -> [_ _ _]
          tunnel: w325 -> [w784 w812 _]
          tunnel: w302 -> [w783 w813 _]
          tunnel: [w782 w811 w839] -> w334
          tunnel: w328 -> [w776 w803 _]
          tunnel: [w781 w810 dbl[][] []] -> w349
          tunnel: w319 -> [w774 w802 _]
          tunnel: [w774 w802 0] -> w318
          event Timeout {
            n285 = event-data() -> ()  [unwired: 1 in, 2 out]
            n286 = local read "Particle Limit"() -> (w777:i64)
            n287 = Array Size(array=w776) -> (size(s)=w780:i32[])
            n288 = Index Array(array=w780, index=0) -> (element=w778:i32)
            n289 = Greater?(x=w778, y=w777) -> (0:w775:bool)
            n290 = case shown="True" w775 {
              tunnel: w784 -> [_ w797]
              tunnel: w783 -> [w786 w792]
              tunnel: [w786 w791] -> w782
              tunnel: w776 -> [w785 w790]
              tunnel: [w785 w787] -> w781
              frame False {
              }
              frame True {
                n291 = Delete From Array(array=w790, index (row)=0) -> (deleted portion=w788:dbl[], array with subset deleted=w787:dbl[][])  [unwired: 2 in]
                n292 = Index Array(array=w788, index=0) -> (element=w798:dbl)
                n293 = Index Array(array=w788, index=1) -> (element=w799:dbl)
                n294 = Search 1D Array(1D array=w797, element=w798) -> (index of element=w793:i32)  [unwired: 1 in]
                n295 = Search 1D Array(1D array=w797, element=w799) -> (index of element=w794:i32)  [unwired: 1 in]
                n296 = Index Array(array=w792, index (row)=w793, index (col)=w794) -> (element=w796:dbl)
                n297 = Decrement(x=w796) -> (x-1=w795:dbl)
                n298 = Replace Array Subset(array=w792, new element=w795, index (row)=w793, index (col)=w794) -> (w791:dbl[][])
              }
            }
          }
          event "Particle Limit": Value Change {
            n299 = event-data() -> ()  [unwired: 1 in, 2 out]
            n300 = Array Size(array=w803) -> (size(s)=w809:i32[])
            n301 = Index Array(array=w809, index=0) -> (element=w807:i32)
            n302 = Greater?(x=w807, y="Particle Limit") -> (0:w804:bool)
            n303 = Subtract(x=w807, y="Particle Limit") -> (x-y=w805:i64)
            n304 = case shown="True" w804 {
              tunnel: w813 -> [w815 w819]
              tunnel: w803 -> [w814 w821]
              tunnel: w812 -> [_ w820]
              tunnel: [w814 w818] -> w810
              tunnel: [w815 w817] -> w811
              tunnel: w805 -> [_ w816]
              frame False {
              }
              frame True {
                n305 = for {
                  N: w816 -> [_]
                  tunnel: w820 -> [w826]
                  shift-right: [w822] -> w817
                  shift-left: w819 -> [w825]
                  shift-right: [w823] -> w818
                  shift-left: w821 -> [w827]
                  n306 = Delete From Array(array=w827, index (row)=0) -> (deleted portion=w824:dbl[], array with subset deleted=w823:dbl[][])  [unwired: 2 in]
                  n307 = Index Array(array=w824, index=0) -> (element=w833:dbl)
                  n308 = Index Array(array=w824, index=1) -> (element=w834:dbl)
                  n309 = Search 1D Array(1D array=w826, element=w833) -> (index of element=w829:i32)  [unwired: 1 in]
                  n310 = Search 1D Array(1D array=w826, element=w834) -> (index of element=w830:i32)  [unwired: 1 in]
                  n311 = Index Array(array=w825, index (row)=w829, index (col)=w830) -> (element=w832:dbl)
                  n312 = Decrement(x=w832) -> (x-1=w831:dbl)
                  n313 = Replace Array Subset(array=w825, new element=w831, index (row)=w829, index (col)=w830) -> (w822:dbl[][])
                }
              }
            }
          }
          event "Clear Spot/Track": Value Change {
            w840 = 49 ("dimension size")
            n314 = event-data() -> ()  [unwired: 1 in, 2 out]
            n315 = local write "Clear Spot/Track"(FALSE ("Clear Spot/Track")) -> ()
            n316 = Initialize Array(0.0 ("element"), w840, w840) -> (w839:dbl[][])
          }
        }
        n317 = case shown="True" "Save Spot Image" {
          tunnel: w274 -> [w759 w769]
          tunnel: [w759 w768] -> w275
          frame False {
          }
          frame True {
            n318 = Format Into String(format string="%03d", initial string="Image", w769) -> (resulting string=w765:string)  [unwired: 1 in, 1 out]
            n319 = Concatenate Strings(w765, ".png" ("string")) -> (w766:string)
            n320 = Build Path(base path="Spot Save Folder", name or relative path=w766) -> (appended path=w767:path)
            n321 = invoke on="Intensity Graph" class="IntGraph (strict)" method="Get Image"("image depth"=32 ("Image Depth")) -> ("image data"=w763:T8)  [unwired: 5 in, 5 out]
            n322 = call <vilib>:"Check if File or Folder Exists.vi"("path"="Spot Save Folder") -> ("file or folder exists?"=w760:bool)  [unwired: 8 in, 2 out]
            n323 = Increment(x=w769) -> (x+1=w768:i32)
            n324 = case shown="True" w760 {
              tunnel: w767 -> [_ w773]
              tunnel: w763 -> [_ w772]
              frame False {
              }
              frame True {
                n325 = call <vilib>:"Write PNG File.vi"("image data"=w772, "path to PNG file"=w773) -> ()  [unwired: 8 in, 2 out]
              }
            }
          }
        }
        n326 = for {
          tunnel: w334 -> [w917] mode=indexing
          tunnel: [w915] -> w371 mode=indexing
          tunnel: [w914] -> w370 mode=indexing
          i -> [w916]
          n327 = for {
            tunnel: w917 -> [w919] mode=indexing
            tunnel: w916 -> [w922]
            tunnel: [w920] -> w914 mode=indexing
            tunnel: [w918] -> w915 mode=indexing
            i -> [w921]
            n328 = Multiply(x=w919, y=w922) -> (x*y=w918:dbl)
            n329 = Multiply(x=w919, y=w921) -> (x*y=w920:dbl)
          }
        }
        n330 = Add Array Elements(numeric array=w334) -> (sum=w337:dbl)
        "# of Particles\nin Spot" <- w337
        n331 = Add Array Elements(numeric array=w371) -> (sum=w369:dbl)
        n332 = Add Array Elements(numeric array=w370) -> (sum=w368:dbl)
        n333 = Divide(x=w369, y=w337) -> (x/y=w367:dbl)
        n334 = Divide(x=w368, y=w337) -> (x/y=w366:dbl)
        n335 = Subtract(x=w367, y=24.0) -> (x-y=w360:dbl)
        n336 = Subtract(x=w366, y=24.0) -> (x-y=w364:dbl)
        n337 = Divide(x=w360, y=2.0) -> (x/y=w305:dbl)
        n338 = Divide(x=w364, y=2.0) -> (x/y=w304:dbl)
        n339 = property on="Intensity Graph" class="IntGraph (strict)"(error in=w307, "Active Cursor"=u32 0, "Cursor.Cursor X"=w305, "Cursor.Cursor Y"=w304) -> (error out=w306:errorcluster)  [unwired: 1 in, 1 out]
        n340 = Build Array(w305, w304) -> (w348:dbl[])
        "Current Spot Pos" <- w348
        n341 = case shown="True" "Load old position\nto Orange Cursor" {
          tunnel: [w904 w909] -> w333
          tunnel: w361 -> [w904 w906]
          tunnel: w286 -> [w903 w911]
          tunnel: [w903 w910] -> w329
          frame False {
          }
          frame True {
            # "DCS DB loading stuff"
            n342 = call <userlib>:"querey dcs spot.vi"("error in (no error)"=w911) -> ("Spot"=w905:T3, "Cancel loading"=w908:bool, "error out"=w910:errorcluster)  [unwired: 15 in, 1 out]
            n343 = Unbundle By Name(w905) -> ("Spot X"=w913:dbl, "Spot Y"=w912:dbl)
            n344 = Build Array(w913, w912) -> (w907:dbl[])
            n345 = Select(t=w906, s=w908, f=w907) -> (s? t:f=w909:dbl[])
          }
        }
        n346 = case shown="False" w314 {
          tunnel: w350 -> [w855 w889]
          tunnel: [w855 w857] -> w347
          tunnel: w302 -> [_ w870]
          tunnel: w338 -> [w854 w869]
          tunnel: w348 -> [_ w867]
          tunnel: [w854 w868] -> w346
          tunnel: w337 -> [_ w861]
          tunnel: [w853 w860] -> w336
          tunnel: w307 -> [w853 w858]
          tunnel: w315 -> [_ w856]
          frame False {
          }
          frame True {
            w880 = sgl 0.0 ("element")
            w881 = sgl 2.0 ("element")
            # "DCS Spots DB stuff"
            n347 = Build Array (concatenate)(w869, w867) -> (w868:dbl[][])
            n348 = Array Max & Min(array=w870) -> (max value=w883:dbl, max index (indices)=w882:i32[])  [unwired: 2 out]
            n349 = Array Size(array=w870) -> (size(s)=w886:i32[])
            n350 = Index Array(array=w867) -> (element #1=w866:dbl, element #2=w865:dbl)  [unwired: 2 in]
            n351 = Multiply Array Elements(1:w886) -> (0:w887:i32)
            n352 = To Variant(anything=w886) -> (Variant=w885:variant)
            n353 = Build Array (concatenate)(w883, w882, w881, w881, w880, w880) -> (w879:dbl[])
            n354 = Reshape Array(w870, w887) -> (w884:dbl[])
            n355 = vi-ref <userlib>:"2DGaussianRotationModelwithOffset.vi"() -> (w888:refnum<vi>)
            n356 = call-poly <vilib>:"Nonlinear Curve Fit.vi"("Y"=w884, "f(x,a)"=w888, "data"=w885, "initial parameters"=w879, "error in (no error)"=w858, "termination"=cluster{"max iteration":i32, "tolerance":dbl} {"max iteration"=1000, "tolerance"=1e-08}) -> ("best fit parameters"=w872:dbl[], "error out"=w859:errorcluster)  [unwired: 4 in, 4 out]
            n357 = Array Subset(array=w872, index=3, length=2) -> (w875:dbl[])
            n358 = Divide(x=24.0 ("y"), y=49.0) -> (x/y=w871:dbl)
            n359 = Multiply(x=w875, y=w871) -> (x*y=w864:dbl[])
            "Spot Widths" <- w864
            n360 = Build Array (concatenate)(w889, w864) -> (w857:dbl[][])
            n361 = Index Array(array=w864) -> (element #1=w863:dbl, element #2=w862:dbl)  [unwired: 2 in]
            n362 = case shown="True" w856 {
              tunnel: w866 -> [_ w898]
              tunnel: w865 -> [_ w897]
              tunnel: w863 -> [_ w896]
              tunnel: w862 -> [_ w895]
              tunnel: w861 -> [_ w894]
              tunnel: [w890 w892] -> w860
              tunnel: w859 -> [w890 w891]
              frame False {
              }
              frame True {
                n363 = Get Date/Time In Seconds() -> (seconds since 1Jan1904=w899:timestamp)
                n364 = call <userlib>:"timestamp_conversion.vi"("error in (no error)"=w891, "Time Stamp"=w899) -> ("error out"=w893:errorcluster, "Integer Time"=w902:i64)  [unwired: 7 in]
                n365 = Bundle By Name(cluster=T3 {"DCS spot ID"=0, "Integer Timestamp"=2, "Spot X"=3.0, "Spot Y"=4.0, "Spot Width X"=0.0, "Spot Width Y"=0.0, "Spot Size"=0, "Experiment Settings ID"=0} ("dcs_spot"), "Integer Timestamp"=w902, "Spot X"=w898, "Spot Y"=w897, "Spot Width X"=w896, "Spot Width Y"=w895, "Spot Size"=w894) -> (w901:T3)
                n366 = call <userlib>:"post_dcs_spot.vi"("error in (no error)"=w893, "dcs_spot"=w901) -> ("error out"=w892:errorcluster)  [unwired: 9 in]
              }
            }
          }
        }
        n367 = Subtract(x="Orange Cursor Position", y=w348) -> (x-y=w343:dbl[])
        n368 = Select(t=w333, s="Load old position\nto Orange Cursor", f=w348) -> (s? t:f=w311:dbl[])
        n369 = Multiply(x=w343, y=8.6106) -> (x*y=w341:dbl[])
        n370 = Or(x="Load old position\nto Orange Cursor", y="Set Orange Cursor\nto current position") -> (x .or. y?=w310:bool)
        n371 = case shown="True" w310 {
          tunnel: "Orange Cursor Position" -> [w751 _]
          tunnel: w311 -> [_ w758]
          tunnel: 1 -> [w748 w756]
          tunnel: w306 -> [w747 w753]
          tunnel: [w746 w752] -> w308
          frame False {
            n372 = Index Array(array=w751) -> (element #1=w750:dbl, element #2=w749:dbl)  [unwired: 2 in]
            n373 = property on="Intensity Graph" class="IntGraph (strict)"(error in=w747, "Active Cursor"=w748, "Cursor.Cursor X"=w750, "Cursor.Cursor Y"=w749) -> (error out=w746:errorcluster)  [unwired: 1 in, 1 out]
          }
          frame True {
            n374 = Index Array(array=w758) -> (element #1=w755:dbl, element #2=w754:dbl)  [unwired: 2 in]
            n375 = local write "Set Orange Cursor\nto current position"(FALSE ("Set Orange Cursor\nto current position")) -> ()
            n376 = local write "Orange Cursor Position"(w758) -> ()
            n377 = property on="Intensity Graph" class="IntGraph (strict)"(error in=w753, "Active Cursor"=w756, "Cursor.Cursor X"=w755, "Cursor.Cursor Y"=w754) -> (error out=w752:errorcluster)  [unwired: 1 in, 1 out]
          }
        }
        n378 = Divide(x=w341, y=2.0) -> (x/y=→"Laser spot\nMove (mm)":dbl[])
        n379 = local read "Tab Control"() -> (w296:T1)
        n380 = local read "Tab Control"() -> (w313:T1)
        n381 = Equal?(x=w296, y=T1."DCS") -> (x = y?=w295:bool)
        n382 = Equal?(x=w313, y=T1."Spot Size Tracking") -> (x = y?=w298:bool)
        n383 = case shown="True" w295 {
          tunnel: w346 -> [_ w743]
          tunnel: w336 -> [w733 w742]
          tunnel: [w733 w741] -> w335
          frame False {
          }
          frame True {
            n384 = Index Array(array=w743, index (col)=0 ("disabled index (col)")) -> (element=w737:dbl[])  [unwired: 1 in]
            n385 = Index Array(array=w743, index (col)=1 ("disabled index (col)")) -> (element=w735:dbl[])  [unwired: 1 in]
            n386 = call "Convert to Dynamic Data"("Array"=w737) -> ("Dynamic Data Type"=w736:dynamicdata)  [unwired: 3 in]
            n387 = call "Convert to Dynamic Data2"("Array"=w735) -> ("Dynamic Data Type"=w734:dynamicdata)  [unwired: 3 in]
            n388 = call "Build XY Graph"("error in (no error)"=w742, "Y Input"=w734, "X Input"=w736) -> ("error out"=w741:errorcluster, "XY Graph"=→"XY Graph":cluster{"Y":dbl[], "Y":dbl[]}[])  [unwired: 2 in, 5 out]
          }
        }
        n389 = case shown="True" w298 {
          tunnel: w347 -> [_ w745]
          frame False {
          }
          frame True {
            n390 = Transpose 2D Array(2D array=w745) -> (transposed array=→"Spot Size over time":dbl[][])
          }
        }
        n391 = Merge Errors(w335, w308, w329) -> (w324:errorcluster)
        "Running Errors" <- w286
      }
      n392 = Not(x=w47) -> (.not. x?=w41:bool)
      n393 = Not Equal To 0?(x=w42) -> (x != 0?=w39:bool)
      n394 = And(x=w39, y=w41) -> (x .and. y?=w40:bool)
      n395 = case shown="True" w40 {
        tunnel: w55 -> [_ w249]
        tunnel: w46 -> [_ w245]
        frame False {
        }
        frame True {
          # "Stuff to post last spot on shutdown"
          n396 = Index Array(array=w249) -> (element #1=w248:dbl, element #2=w247:dbl)  [unwired: 2 in]
          n397 = Array Size(array=w245) -> (size(s)=w246:i32[])
          n398 = local read "# of Particles\nin Spot"() -> (w239:dbl)
          n399 = Get Date/Time In Seconds() -> (seconds since 1Jan1904=w253:timestamp)
          n400 = Index Array(array=w246) -> (element=w244:i32)  [unwired: 1 in]
          n401 = call <userlib>:"timestamp_conversion.vi"("Time Stamp"=w253) -> ("Integer Time"=w252:i64)  [unwired: 8 in, 1 out]
          n402 = Index Array(array=w245, index (row) #1=w244, index (col) #1=0 ("disabled index (col)"), index (row) #2=w244, index (col) #2=1 ("disabled index (col)")) -> (element #1=w243:dbl, element #2=w240:dbl)
          n403 = Bundle By Name(cluster=T3 {"DCS spot ID"=0, "Integer Timestamp"=2, "Spot X"=3.0, "Spot Y"=4.0, "Spot Width X"=0.0, "Spot Width Y"=0.0, "Spot Size"=0, "Experiment Settings ID"=0} ("dcs_spot"), "Integer Timestamp"=w252, "Spot X"=w248, "Spot Y"=w247, "Spot Width X"=w243, "Spot Width Y"=w240, "Spot Size"=w239) -> (w250:T3)
          n404 = call <userlib>:"post_dcs_spot.vi"("dcs_spot"=w250) -> ()  [unwired: 10 in, 1 out]
        }
      }
    }
    frame Error {
    }
  }
  "error out" <- w13
